vi "placeholder--create.vi"(11 "TEMPLATE Actor in":refnum<class "TEMPLATE Actor.lvclass">) -> (0 "Error out":errorcluster, 3 "TEMPLATE Actor out":refnum<class "TEMPLATE Actor.lvclass">)   [LabVIEW 2025, in "TEMPLATE Actor.lvlib" / "TEMPLATE Actor.lvclass"]
uses:
  TEMPLATE Actor.lvclass
  C:/Program Files/National Instruments/LabVIEW 2025/vi.lib/Nathan Davis/jettl/jettl/jettl/Actor/Actor/Actor.lvclass
  <vilib>/Nathan Davis/jettl/jettl/jettl/Actor/Actor.lvlib
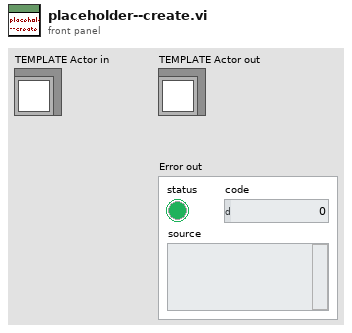
[diagram p1: front panel]
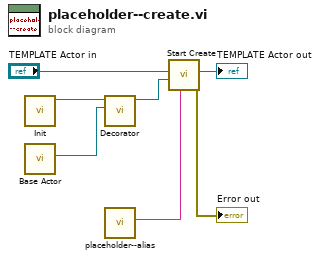
[diagram p0: block diagram]
diagram:
  n1 = call "Init.vi"() -> ("TEMPLATE Actor out"=w5:refnum<class "TEMPLATE Actor.lvclass">)  [unwired: 11 in]
  n2 = call <vilib>:"Base Actor.vi"() -> ("Actor"=w4:refnum<class "Actor.lvclass">)  [unwired: 11 in]
  n3 = call-dynamic "Decorator.vi"("Actor"=w4, "TEMPLATE Actor in"=w5) -> ("TEMPLATE Actor out"=w3:refnum<class "TEMPLATE Actor.lvclass">)  [unwired: 9 in]
  n4 = call "placeholder--alias.vi"() -> ("Prefix"=w2:string)  [unwired: 11 in]
  n5 = call <vilib>:"Start Create.vi"("Alias"=w2, "Actor"=w3, "Actor in"="TEMPLATE Actor in") -> ("Error out"=→"Error out":errorcluster, "Actor out"=→"TEMPLATE Actor out":refnum<class "TEMPLATE Actor.lvclass">)  [unwired: 7 in]
